vi "Open.vi"(8 "error in (no error)":errorcluster caption="entrée d'erreur (pas d'erreur)", 11 "Class Multimeter Rigol DM3058 en entrée":refnum<class "Class Multimeter Rigol DM3058.lvclass">) -> (0 "error out":errorcluster caption="sortie d'erreur", 3 "Class Multimeter Rigol DM3058 en sortie":refnum<class "Class Multimeter Rigol DM3058.lvclass">)   [LabVIEW 2020, in "Library Instrument & Equipement.lvlib" / "Library Multimeter.lvlib" / "Class Multimeter Rigol DM3058.lvclass"]
uses:
  Class Multimeter Rigol DM3058.lvclass
  C:/Users/ngarcin/OneDrive - Altyor/Standard TB/Class/Multimeter/Multimeter (Default)/Class Multimeter (Default).lvclass
  Commun VI/TypeDef/Liste Error.ctl
  Class Multimeter Rigol DM3058.lvclass/Class Multimeter Rigol DM3058.ctl
  RIGOL DM3058/RIGOL DM3058.lvlib
  Commun VI/Library Commun.lvlib
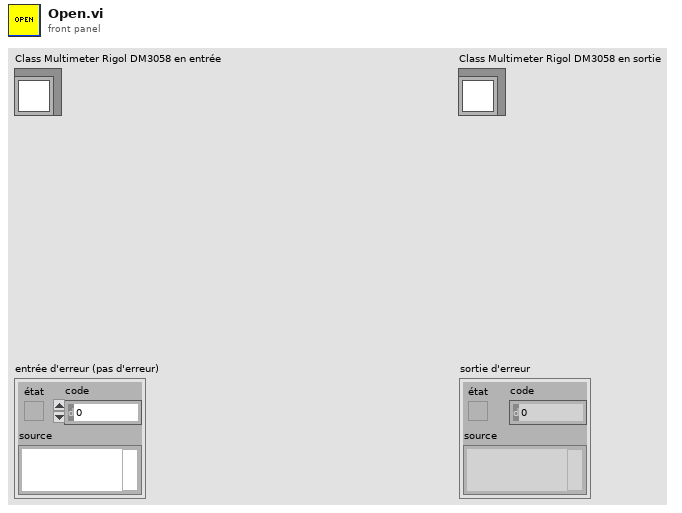
[diagram p1: front panel]
types:
  T1 = typedef "Library Commun.lvlib/Liste Error.ctl" = enum16{"Firebase Driver - Get Document", "Firebase Driver - Get Document With Where", "Firebase Driver - Delete Document", "Firebase Driver - Set Document", "Firebase Driver - Update Document", "Firebase Altyor - Search Document Bench", "Firebase Altyor - Class Not in Firebase", "Spectrum_Analyser - Timeout", "Relay Board - Qty Relay", "DIO - Pb Funtion", "Power_Supply - Peripherical not find", "Mutimeter - Peripherical not find", "Instrument - Function Not Used", "Instrument - Instrument name not specified", "Instrument - Allready Initialised", "Instrument - TimeOut", "Instrument - the instrument must be Initialise before", "Instrument - Frame Not received", "Instrument - Frame Nok", "Test - Initialise the File_for_Save", "Test - Timeout", "Test - Cmd Error", "FGV - Variable ", "BDD FireBase - Define Class", "SN - Class Not Define"}
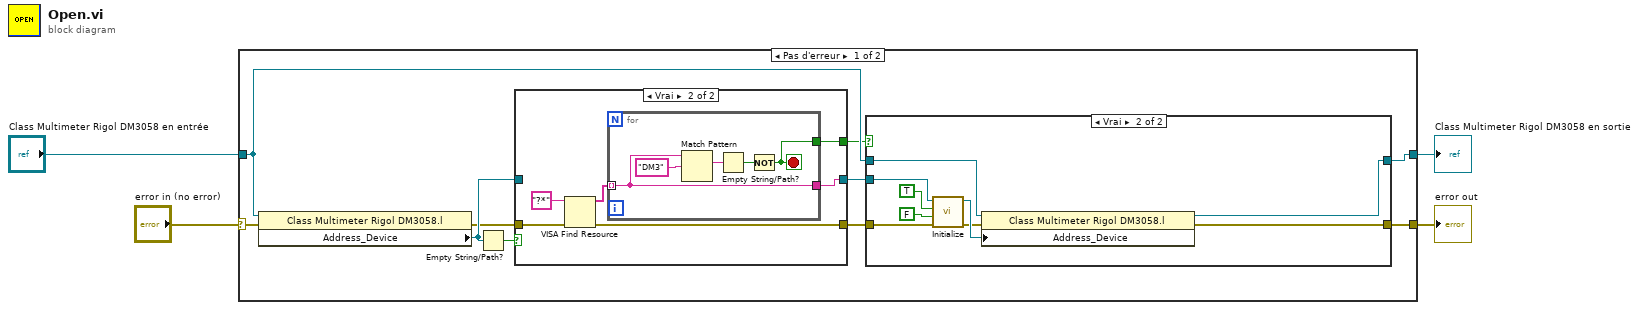
[diagram p0: block diagram]
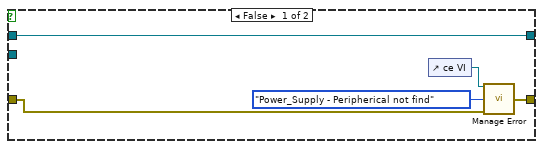
[diagram p2: hidden frame]
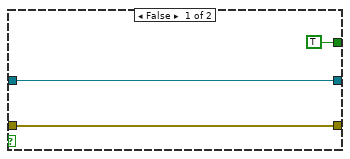
[diagram p3: hidden frame]
diagram:
  n1 = case shown="Pas d'erreur" "error in (no error)" {
    selector: "error in (no error)" -> [w14 w44]
    tunnel: "Class Multimeter Rigol DM3058 en entrée" -> [w13 w43]
    tunnel: [w6 w44] -> w2
    tunnel: [w5 w43] -> w1
    frame No Error {
      n2 = property class="Class Multimeter Rigol DM3058.l"(reference=w13, error in=w14) -> (error out=w9:errorcluster, "Address_Device"=w11:refnum<visa-resource-name>)  [unwired: 1 out]
      n3 = Empty String/Path?(string/path=w11) -> (empty?=w12:bool)
      n4 = case shown="Vrai" w12 {
        tunnel: [TRUE w35] -> w7
        tunnel: [w30 w34] -> w10
        tunnel: w11 -> [w30 _]
        tunnel: w9 -> [w29 w33]
        tunnel: [w29 w32] -> w8
        frame False {
        }
        frame True {
          n5 = VISA Find Resource(8:w33, 11:"?*" ("expression  (\"?*\")")) -> (0:w32:errorcluster, 3:w36:string[])  [unwired: 1 in, 1 out]
          n6 = for {
            tunnel: w36 -> [w39] mode=indexing
            tunnel: [w39] -> w34
            tunnel: [w38] -> w35
            stop <- w38 stop-if-true
            n7 = Match Pattern(string=w39, regular expression="DM3" ("expression régulière")) -> (match substring=w41:string)  [unwired: 1 in, 3 out]
            n8 = Empty String/Path?(string/path=w41) -> (empty?=w40:bool)
            n9 = Not(x=w40) -> (.not. x?=w38:bool)
          }
        }
      }
      n10 = case shown="Vrai" w7 {
        tunnel: w13 -> [w17 w26]
        tunnel: [w16 w23] -> w6
        tunnel: [w17 w22] -> w5
        tunnel: w10 -> [_ w21]
        tunnel: w8 -> [w15 w20]
        frame False {
          n11 = control-ref of="ce VI"() -> (w19:refnum<vi>)
          n12 = call "Manage Error.vi"("VI in Error"=w19, "Code Erreur"=Liste_Error."Power_Supply - Peripherical not find", "error in (no error)"=w15) -> ("error out"=w16:errorcluster)  [unwired: 12 in]
        }
        frame True {
          n13 = call "Initialize.vi"("error in (no error)"=w20, "Reset (True)"=FALSE, "ID Query (True)"=TRUE, "VISA resource name"=w21) -> ("error out"=w24:errorcluster, "VISA resource name out"=w25:refnum<visa-resource-name>)  [unwired: 6 in]
          n14 = property class="Class Multimeter Rigol DM3058.l"(reference=w26, error in=w24, "Address_Device"=w25) -> (reference out=w22:refnum<class "Class Multimeter Rigol DM3058.lvclass">, error out=w23:errorcluster)
        }
      }
    }
    frame Error {
    }
  }
  "error out" <- w2
  "Class Multimeter Rigol DM3058 en sortie" <- w1
